vi "moveBoom (SubVI).vi"(11 "Boom stoke(mm)":sgl) -> (3 "Boom angle(deg)":sgl)   [LabVIEW 2020]
uses:
  <vilib>/imath/engines/lvmath2/RunTimeEngine/NodeEndStatement/NIMS_NodeEndStatement_Output.vi
  <instcachedir>/0/NIMS_NodeEndStatement_Output_53EC0D466D134D7ABD903AC30B43404B.lvgen/NIMS_NodeEndStatement_Output_53EC0D466D134D7ABD903AC30B43404B_009.vi
  <vilib>/imath/engines/lvmath2/RunTimeEngine/ErrorHandling/NIMS_Finalize Error.vi
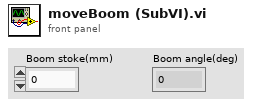
[diagram p1: front panel]
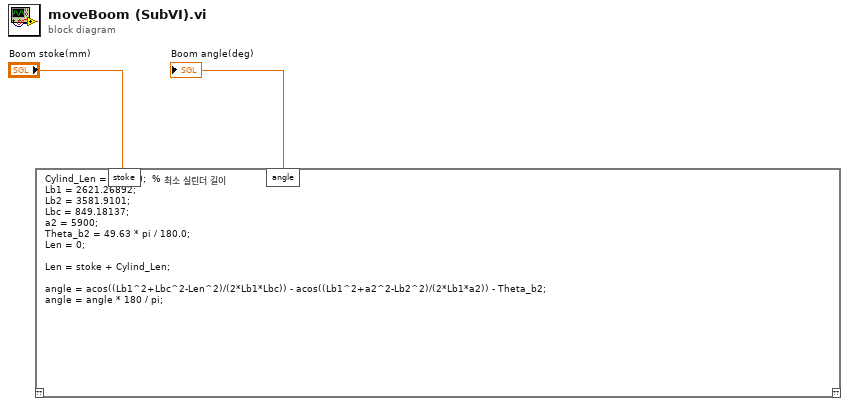
[diagram p0: block diagram]
diagram:
  n1 = mathscript code="Cylind_Len = 1885.0;  % 최소 실린더 길이\nLb1 = 2621.26892;\nLb2 = 3581.9101;\nLbc = 849.18137;\na2 = 5900;\nTheta_b2 = 49.63 * pi / 180.0;\nLen = 0;\n\nLen = stoke + Cylind_Len;\n\nangle = acos((Lb1^2+Lbc^2-Len^2)/(2*Lb1*Lbc)) - acos((Lb1^2+a2^2-Lb2^2)/(2*Lb1*a2)) - Theta_b2;\nangle = angle * 180 / pi;"("stoke"="Boom stoke(mm)") -> ("angle"=→"Boom angle(deg)":cdb)  [unwired: 1 in, 1 out]
